vi "Process Name.vi"() -> (3 "process name":string)   [LabVIEW 2021, in "AudioGenTCPReaderProcess.lvlib"]
uses:
  AudioGenTCPReaderProcess.lvlib
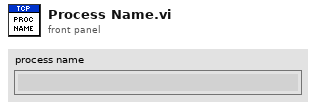
[diagram p1: front panel]
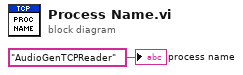
[diagram p0: block diagram]
diagram:
  "process name" <- "AudioGenTCPReader" ("ProcessName")
